vi "Init Ball Loading Screen.vi"(11 "AllObjs[]":refnum<vi>[](array[refnum])) -> (2 "Array 2":refnum<vi>[](array[refnum]), 3 "Array":i32[](array[numeric]))   [LabVIEW 2014, in "Endigit.lvlib"]
uses:
  Endigit.lvlib
panel:
  # "https://decibel.ni.com/content/docs/DOC-1086"
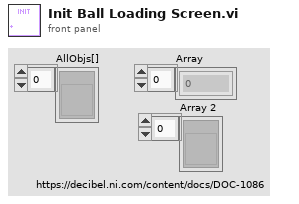
[diagram p1: front panel]
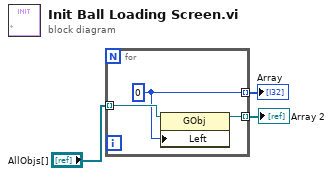
[diagram p0: block diagram]
diagram:
  n1 = for {
    tunnel: "AllObjs[]" -> [w6] mode=indexing
    tunnel: [w5] -> w3 mode=indexing
    tunnel: [w4] -> w1 mode=indexing
    w5 = 0 ("y")
    n2 = property class="GObj"(reference=w6, "Left"=w5) -> (reference out=w4:refnum<vi>)  [unwired: 1 in, 1 out]
  }
  "Array" <- w3
  "Array 2" <- w1
